vi "DelayFind.vi"() -> ()   [LabVIEW 2020]
doc: "Example Description:\nThis example demonstrates how to enable Time Interleaved Sampling with the NI 5772 adapter module to achieve a sampling rate of 1.6GS/s. This example continuously acquires records of analog input data from the NI 5772 adapter module. It allows you to select an AI channel, trigger type, and record size. This VI must be compiled before it is run. \n\nVI Configuration:\nThis example uses the NI PXI-7952R as the FPGA target by default. If you are using another FPGA target, complete the following steps to configure the host VI to use a VI configured for your FPGA target:\n1. On the block diagram, right-click the Open FPGA VI Reference (NI PXI-7952R) function and select Configure Open FPGA VI Reference.\n2. Browse for a new target by clicking the Browse Project button in the Open VI section.\n3. Select the VI under the target that matches your device. Click OK to select this VI.\n4. Click OK to exit the dialog box and to apply the new selection to the FPGA VI.\n5. Save the VI.\n\nRunning the VI:\n1. Select a RIO Resource that corresponds to the FPGA device configured above.\n2. Clock Configuration: Select the desired clock source for the adapter module.\nAnalog Input: Configure the AI Channel, Record Size, and Trigger Type controls. If you are using the analog trigger type, configure the Trigger Level (V) control.\n3. Click the run arrow to run the VI.\n4. If the Trigger Type is set to Software, click the Software Trigger button to acquire a single record of data. If the Trigger Type is set to Data Edge, a record of data is acquired each time the input signal rises above the trigger level.\n\nThe Record Size, Trigger Type, and Trigger Level (V) controls can all be configured while the VI is running. \n\nNote: The AI Channel control must be configured before the VI is run.\n\nExecution Steps:s\n1. Open a session to the FPGA VI and run the VI.\n2. Wait for the adapter module to load its default configuration.\n3. Configure the NI 5772 for Time Interleaved Sampling (TIS)\n4. The Trigger type and record size for a single record acquisition are configured.\n5. Based on the trigger type, either wait for the software trigger Boolean to assert or configure the desired trigger level and arm the trigger.\n6. After the trigger is armed, a single record of data is acquired and read.\n7. Stop the VI when the stop button is pressed or when an error has occurred. \n8. Close the FPGA VI reference and display any errors."
uses:
  <vilib>/userDefined/High Color/nirio_resource_hc.ctl
  <vilib>/Utility/error.llb/Error Cluster From Error Code.vi
  <vilib>/rvi/errors/niLvFpgaAdjustHostInterfaceError.vi
  <vilib>/FPGAPlugInAG/Dynamic/niLvFpga_Close_Dynamic.vi
  <vilib>/rvi/interface/nirviReadWriteControl/nirviReadWriteControl.xnode
  SubVIs/DigiFPGARef.ctl
  <vilib>/rvi/interface/nirviCloseFPGA/nirviCloseFPGA.xnode
  NiFpgaLv.dll
  <vilib>/rvi/interface/Simulation/niFpgaSimulationCallBeginRW.vi
  <instrlib>/_niInstr/Basic Elements/v1/FPGA/niInstr Basic Elements v1 FPGA.lvlib
panel:
  in  "Use Default Wave Settings":bool caption="Checkbox"
  in  "Generator Resource":refnum<k15>="PXI1Slot3"
  out "Actual Sample Rate":dbl
  in  "nGenTrig/vi":bool=TRUE caption="Trigger Mode"
  out "TIS Configured?":bool
  in  "RIO Resource":T1="PXI1Slot2"
  out "Configured?":bool
  in  "Ext/nViTrig":bool=TRUE
  in  "stop Gen":bool
  in  "Send vi Trig":bool
  out "Waveform LIVE":waveform(ext)(graph)
  in  "Record Size":u16=1024
  in  "Delay(us)":sgl min=0 step=0.1 format="%#_4g"
  in  "Trigger Level (V)":dbl
  in  "Wave Sampling Rate":sgl=200000000.0
  out "WaveSampleCount":sgl=1024.0
  in  "Time Avg":u8(knob) max=2 step=1 scale=0.0..2.0
  in  "AvgCount_powerOf2":i16(knob) caption="Amplitude Avg" min=0 max=8 step=1 scale=0.0..8.0
  in  "TrigIn_Sim":bool caption="Pause"
  out "error out":errorcluster
  in  "stop":bool caption="Stop"
  in  "Trigger Type":enum8{"Software", "Data Edge"}(ring)
  # "Resource Configuration"
  # "Configuration"
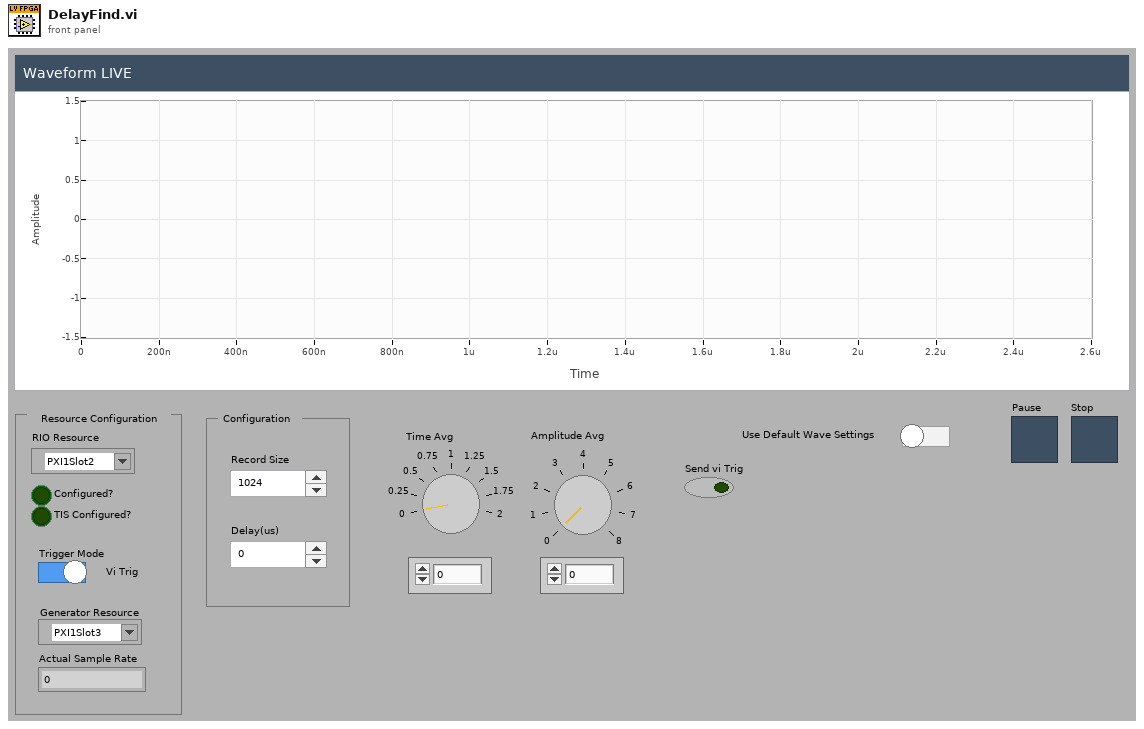
[diagram p1: front panel]
types:
  T1 = typedef "nirio_resource_hc.ctl" = tag
  T2 = typedef "DigiFPGARef.ctl" = refnum<k20>
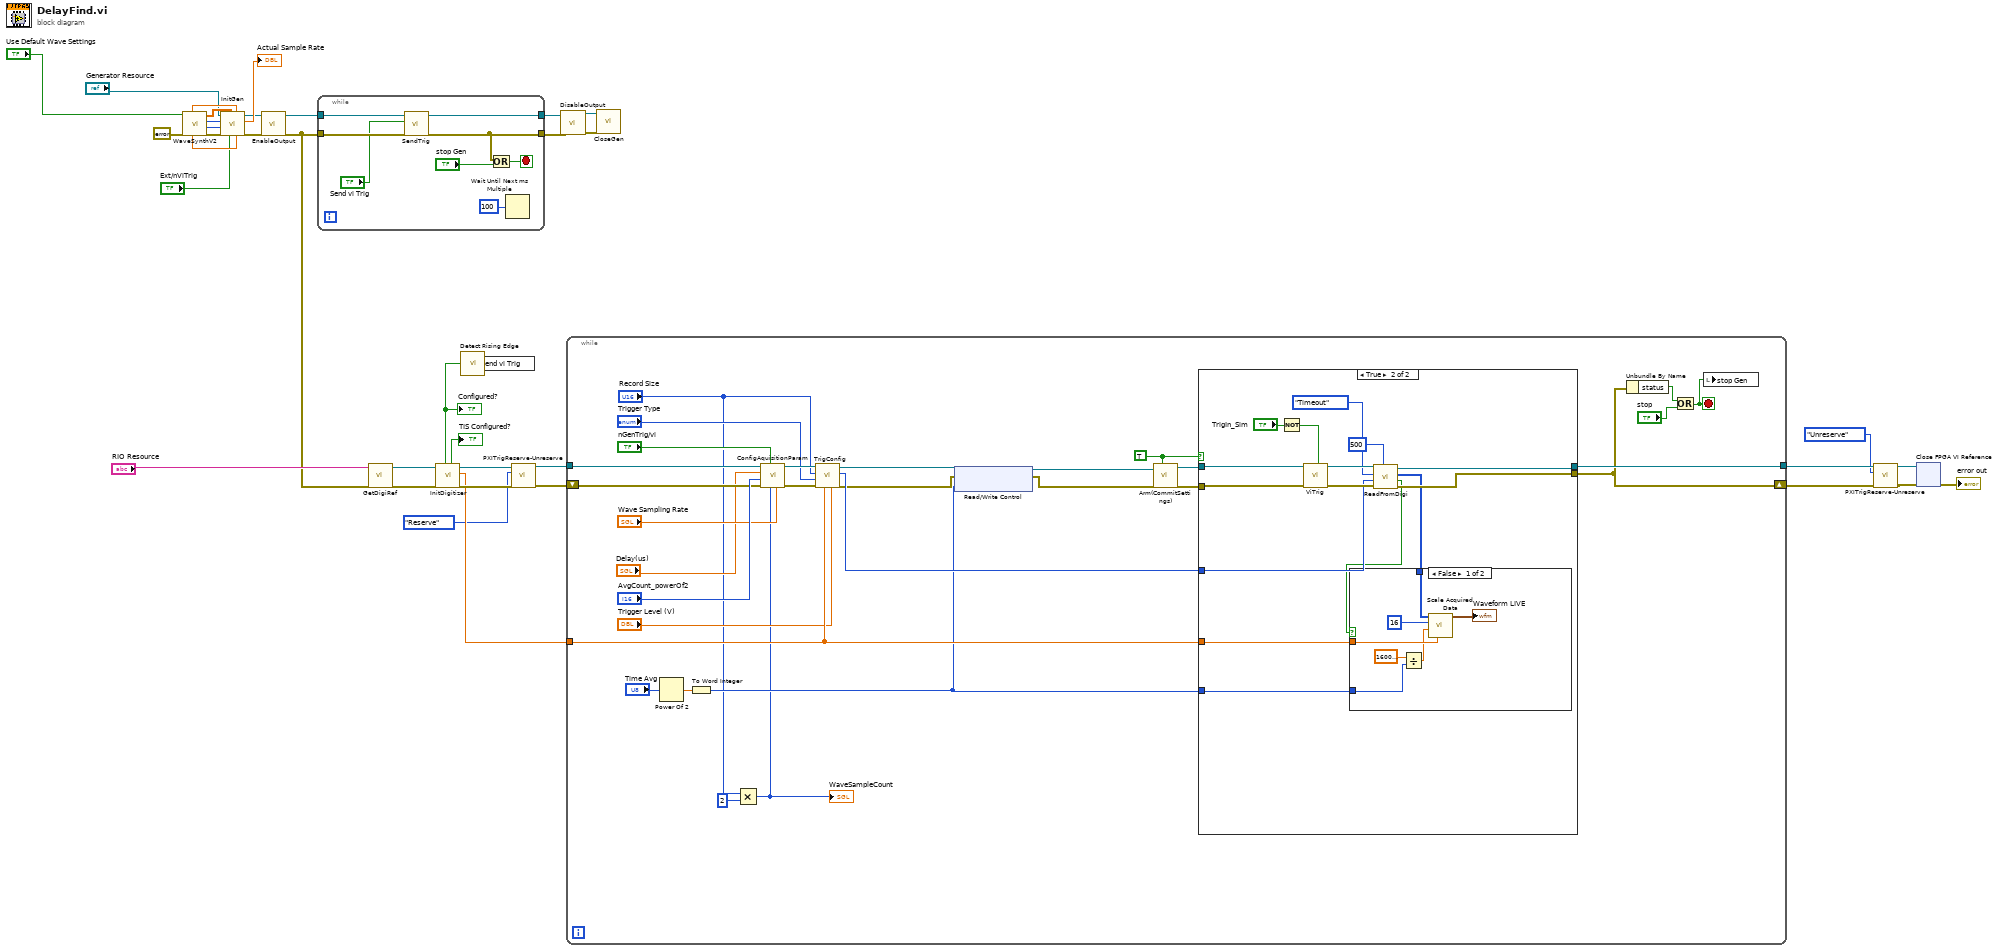
[diagram p0: block diagram]
diagram:
  n1 = call "WaveSynthV2.vi"("error in"=errorcluster {"status"=FALSE, "code"=0, "source"=""}, "Default Wave"="Use Default Wave Settings") -> ("error out"=w7:errorcluster, "Waves per Pixel"=w9:u32, "Sampling Frequency (Hz)"=w11:u64, "Amplitudes"=w10:dbl[], "Offset Factor"=w12:dbl, "Gain"=w13:dbl)  [unwired: 2 in]
  n2 = call "InitGen.vi"("Offset"=w12, "Gain"=w13, "Ext/nViTrig"="Ext/nViTrig", "Waveform Data Array"=w10, "error in (no error)"=w7, "Wave Per Pixel"=w9, "Sample Rate (Samp/s)"=w11, "FGEN Resource Name"="Generator Resource") -> ("error out"=w19:errorcluster, "Actual Sample Rate"=→"Actual Sample Rate":dbl, "reference out"=w20:refnum<k15>)  [unwired: 1 in]
  n3 = call "EnableOutput.vi"("error in (no error)"=w19, "FGEN Resource Name"=w20) -> ("error out"=w5:errorcluster, "Instrument Handle Out"=w18:refnum<k15>)  [unwired: 8 in]
  n4 = while {
    tunnel: w18 -> [w42]
    tunnel: w5 -> [w41]
    tunnel: [w39] -> w14
    tunnel: [w40] -> w15
    stop <- w43 stop-if-true
    n5 = call "SendTrig.vi"("error in (no error)"=w41, "Send vi Trig"="Send vi Trig", "Instrument Handle"=w42) -> ("error out"=w40:errorcluster, "Instrument Handle Out"=w39:refnum<k15>)  [unwired: 7 in]
    n6 = Or(x=w40, y="stop Gen") -> (x .or. y?=w43:bool)
    n7 = Wait Until Next ms Multiple(millisecond multiple=u32 100) -> ()  [unwired: 1 out]
  }
  n8 = call "GetDigiRef.vi"("error in (no error)"=w5, "RIO Device IN"="RIO Resource") -> ("error out"=w36:errorcluster, "FPGA VI Reference Out"=w27:T2)  [unwired: 8 in]
  n9 = call "InitDigitizer.vi"("error in"=w36, "FPGA VI Reference"=w27) -> ("error out"=w33:errorcluster, "range (Vpp)"=w32:dbl, "FPGA VI Reference Out"=w34:T2, "TIS Configured?"=→"TIS Configured?":bool, "Configured?"=w3:bool)  [unwired: 5 in]
  "Configured?" <- w3
  n10 = call <instrlib>:"Detect Rising Edge.vi"("signal"=w3) -> ("edge detected"=w1:bool)  [unwired: 14 in]
  n11 = local write "Send vi Trig"(w1) -> ()
  n12 = call "PXITrigReserve-Unreserve.vi"("error in"=w33, "Mode"=enum16{"Reserve", "Unreserve"}."Reserve", "FPGA VI Reference"=w34) -> ("error out"=w29:errorcluster, "FPGA VI Reference Out"=w30:T2)  [unwired: 7 in]
  n13 = call "DisableOutput.vi"("error in (no error)"=w15, "FGEN Resource Name"=w14) -> ("error out"=w16:errorcluster, "Instrument Handle Out"=w17:refnum<k15>)  [unwired: 8 in]
  n14 = while {
    tunnel: [w57] -> w26
    shift-right: [w56] -> w25
    shift-left: w29 -> [w67]
    tunnel: w32 -> [w65]
    tunnel: w30 -> [w73]
    stop <- w46 stop-if-true
    w61 = TRUE ("Arm?")
    n15 = Power Of 2(x="Time Avg") -> (2^x=w58:dbl)
    n16 = To Word Integer(number=w58) -> (16bit integer=w51:i16)
    n17 = Multiply(x="Record Size", y=u16 2) -> (x*y=w50:u16)
    "WaveSampleCount" <- w50
    n18 = call "ConfigAquisitionParam.vi"("Wave Sampling Rate"="Wave Sampling Rate", "WaveSampleCount"=w50, "vi/nGenTrig"="nGenTrig/vi", "error in"=w67, "AvgCount_powerOf2"="AvgCount_powerOf2", "Delay (us)"="Delay(us)", "FPGA VI Reference"=w73) -> ("error out"=w71:errorcluster, "FPGA VI Reference Out"=w72:T2)  [unwired: 3 in]
    n19 = call "TrigConfig.vi"("Trigger Level (V)"="Trigger Level (V)", "range (Vpp)"=w65, "error in"=w71, "Trigger Type"="Trigger Type", "Requested Samples Per Pixel"="Record Size", "FPGA VI Reference"=w72) -> ("error out"=w54:errorcluster, "Read Size (Host)"=w60:u16, "FPGA VI Reference Out"=w55:T2)  [unwired: 3 in]
    n20 = xnode "Read/Write Control"("FPGA VI Reference In"=w55, "error in"=w54, "Neighbour Avg"=w51) -> ("FPGA VI Reference Out"=w53:T2, "error out"=w52:errorcluster)
    n21 = call "Arm(CommitSettings).vi"("Arm?"=w61, "error in"=w52, "FPGA VI Reference"=w53) -> ("error out"=w62:errorcluster, "FPGA VI Reference Out"=w63:T2)  [unwired: 7 in]
    n22 = case shown="True" w61 {
      tunnel: w63 -> [w76 w82]
      tunnel: w62 -> [w77 w92]
      tunnel: [w77 w88] -> w56
      tunnel: [w76 w89] -> w57
      tunnel: w65 -> [_ w84]
      tunnel: w60 -> [_ w87]
      tunnel: w51 -> [_ w79]
      frame False {
      }
      frame True {
        n23 = Not(x="TrigIn_Sim") -> (.not. x?=w78:bool)
        n24 = call "ViTrig.vi"("Vi Trigger"=w78, "error in"=w92, "FPGA VI Reference"=w82) -> ("error out"=w90:errorcluster, "FPGA VI Reference Out"=w91:T2)  [unwired: 7 in]
        n25 = call "ReadFromDigi.vi"("Timeout (ms)"=500, "error in"=w90, "Number of Elements"=w87, "Mode"=enum16{"Wait For Data", "Timeout"}."Timeout", "FPGA VI Reference"=w91) -> ("error out"=w88:errorcluster, "Error/Timeout?"=w81:bool, "Output Waveform"=w85:u16[], "FPGA VI Reference Out"=w89:T2)  [unwired: 3 in]
        n26 = case shown="False" w81 {
          tunnel: w85 -> [w98 _]
          tunnel: w84 -> [w96 _]
          tunnel: w79 -> [w94 _]
          frame False {
            n27 = Divide(x=1600000000.0 ("Sample Rate"), y=w94) -> (x/y=w95:dbl)
            n28 = call "Scale Acquired Data.vi"("range (V)"=w96, "Sample Rate"=w95, "Number of Bits"=i16 16, "Data In"=w98) -> ("output waveform"=→"Waveform LIVE":waveform(ext))  [unwired: 7 out]
          }
          frame True {
          }
        }
      }
    }
    n29 = Unbundle By Name(w56) -> ("status"=w74:bool)
    n30 = Or(x=w74, y="stop") -> (x .or. y?=w46:bool)
    n31 = local write "stop Gen"(w46) -> ()
  }
  n32 = call "CloseGen.vi"("error in (no error)"=w16, "Instrument Handle"=w17) -> ()  [unwired: 9 in, 1 out]
  n33 = call "PXITrigReserve-Unreserve.vi"("error in"=w25, "Mode"=enum16{"Reserve", "Unreserve"}."Unreserve", "FPGA VI Reference"=w26) -> ("error out"=w22:errorcluster, "FPGA VI Reference Out"=w23:T2)  [unwired: 7 in]
  n34 = xnode "Close FPGA VI Reference"("FPGA VI Reference In"=w23, "error in"=w22) -> ("error out"=→"error out":errorcluster)
